vi "Read from UDP.vi"(8 "error in":errorcluster, 11 "Control Loop Cluster":T1) -> (0 "error out":errorcluster, 3 "Control Loop Cluster Out":T1)   [LabVIEW 2021, in "RT Main.lvlib"]
uses:
  RT Main.lvlib
  Control Loop Cluster.ctl
  <vilib>/myRIO/Instrument Drivers/Onboard IO/AI/typedefs/AI Reference.ctl
  <vilib>/myRIO/Common/Instrument Driver Framework/Utilities/typedefs/myRIO Generic Hardware Reference.ctl
  <vilib>/myRIO/Common/Instrument Driver Framework/Utilities/typedefs/Hardware Version Enum.ctl
  <vilib>/myRIO/Common/Instrument Driver Framework/Utilities/typedefs/myRIO v1.0 Reference.ctl
  <vilib>/myRIO/Common/Instrument Driver Framework/Utilities/typedefs/Generic FPGA Reference.ctl
  <vilib>/myRIO/Common/Instrument Driver Framework/myRIO v1.0/AI/typedefs/AI Channels List.ctl
  <vilib>/myRIO/Common/Instrument Driver Framework/myRIO v1.0/AI/typedefs/AI Channels Enum.ctl
  <vilib>/myRIO/Common/Instrument Driver Framework/Utilities/typedefs/Analog Scaling Constants List.ctl
  <vilib>/myRIO/Common/Instrument Driver Framework/Utilities/typedefs/Analog Scaling Constants.ctl
  <vilib>/myRIO/Instrument Drivers/Onboard IO/DIO/typedefs/DIO Reference.ctl
  <vilib>/myRIO/Common/Instrument Driver Framework/myRIO v1.0/DIO/typedefs/DIO Channels List.ctl
  <vilib>/myRIO/Common/Instrument Driver Framework/myRIO v1.0/DIO/typedefs/DIO Channels Enum.ctl
  Data Cluster.ctl
  Libraries/Common RT/Hardware Monitoring.ctl
  <vilib>/myRIO/Instrument Drivers/Onboard IO/AI/AI.lvlib
  <vilib>/myRIO/Instrument Drivers/Onboard IO/DIO/DIO.lvlib
  Libraries/Common RT/Common RT.lvlib
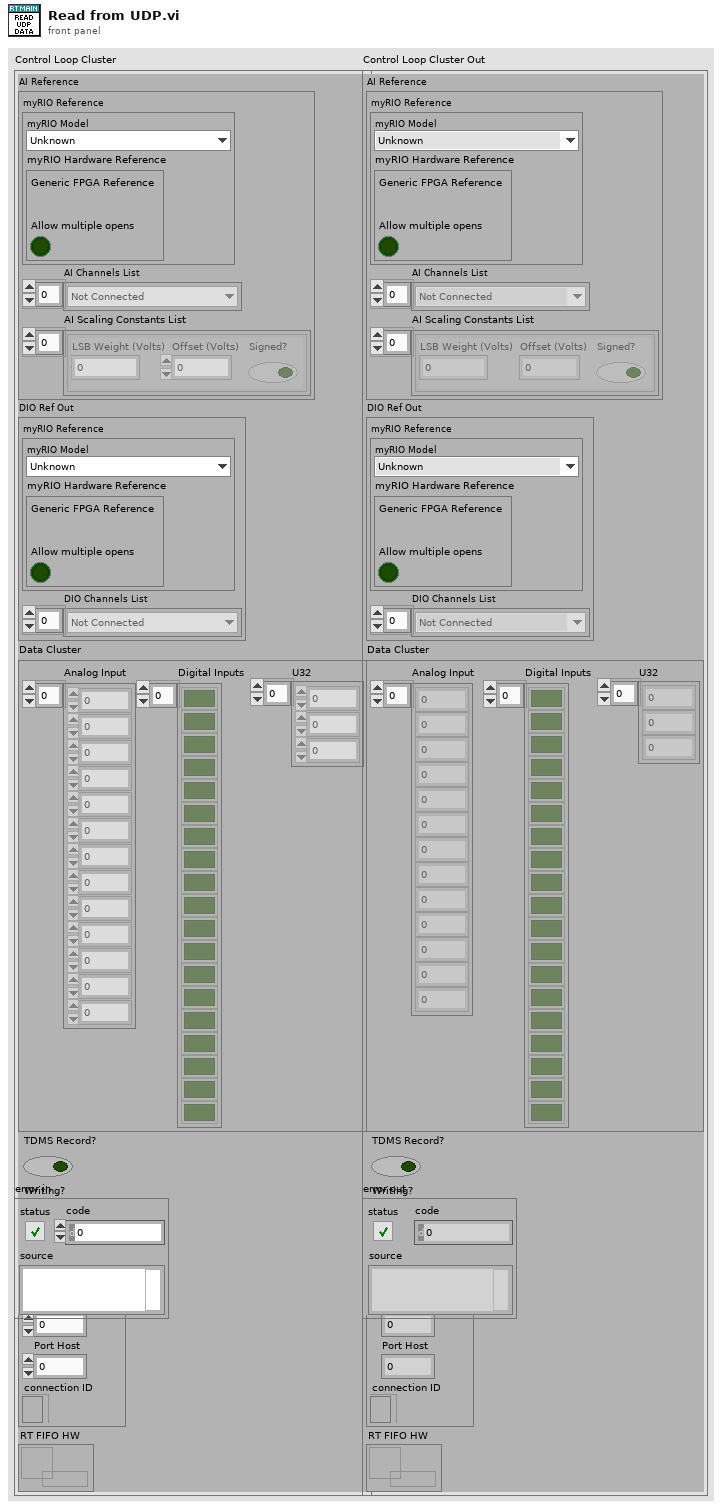
[diagram p1: front panel]
types:
  T1 = typedef "RT Main.lvlib/Control Loop Cluster.ctl" = cluster{"AI Reference":T2, "DIO Reference":T11, "Data Cluster":T14, "TDMS Record?":bool, "Writing?":bool, "UDP Info":cluster{"IP Host":string, "Port RT":u16, "Port Host":u16, "connection ID":refnum<k16>}, "RT FIFO HW":refnum<k33>}
  T2 = typedef "AI.lvlib/AI Reference.ctl" = cluster{"myRIO Reference":T3, "AI Channels List":T7, "AI Scaling Constants List":T9}
  T3 = typedef "myRIO Generic Hardware Reference.ctl" = cluster{"myRIO Model":T4, "myRIO Hardware Reference":T5}
  T4 = typedef "Hardware Version Enum.ctl" = enum16{"Unknown", "myRIO-1900", "myRIO-1950", "roboRIO", "NI ELVIS RIO CM", "ELVIS III"}
  T5 = typedef "myRIO v1.0 Reference.ctl" = cluster{"Generic FPGA Reference":T6, "Allow multiple opens":bool}
  T6 = typedef "Generic FPGA Reference.ctl" = refnum<k20>
  T7 = typedef "AI Channels List.ctl" = T8[]
  T8 = typedef "AI Channels Enum.ctl" = enum16{"Not Connected", "AudioIn/Left", "AudioIn/Right", "C/AI0", "C/AI1", "A/AI0", "A/AI1", "A/AI2", "A/AI3", "A/AI4", "A/AI5", "A/AI6", "A/AI7", "B/AI0", "B/AI1", "B/AI2", "B/AI3", "B/AI4", "B/AI5", "B/AI6", "B/AI7", "AI/AI0", "AI/AI1", "AI/AI2", "AI/AI3", "A/AI0 (DIFF)", "A/AI1 (DIFF)", "A/AI2 (DIFF)", "A/AI3 (DIFF)", "B/AI0 (DIFF)", "B/AI1 (DIFF)", "B/AI2 (DIFF)", "B/AI3 (DIFF)"}
  T9 = typedef "Analog Scaling Constants List.ctl" = T10[]
  T10 = typedef "Analog Scaling Constants.ctl" = cluster{"LSB Weight (Volts)":dbl, "Offset (Volts)":dbl, "Signed?":bool}
  T11 = typedef "DIO.lvlib/DIO Reference.ctl" = cluster{"myRIO Reference":T3, "DIO Channels List":T12}
  T12 = typedef "DIO Channels List.ctl" = T13[]
  T13 = typedef "DIO Channels Enum.ctl" = enum16{"Not Connected", "C/DIO0", "C/DIO1", "C/DIO2", "C/DIO3", "C/DIO4", "C/DIO5", "C/DIO6", "C/DIO7", "A/DIO0", "A/DIO1", "A/DIO2", "A/DIO3", "A/DIO4", "A/DIO5", "A/DIO6", "A/DIO7", "A/DIO8", "A/DIO9", "A/DIO10", "A/DIO11", "A/DIO12", "A/DIO13", "A/DIO14", "A/DIO15", "A/DIO16", "A/DIO17", "A/DIO18", "A/DIO19", "B/DIO0", "B/DIO1", "B/DIO2", "B/DIO3", "B/DIO4", "B/DIO5", "B/DIO6", "B/DIO7", "B/DIO8", "B/DIO9", "B/DIO10", "B/DIO11", "B/DIO12", "B/DIO13", "B/DIO14", "B/DIO15", "B/DIO16", "B/DIO17", "B/DIO18", "B/DIO19", "LED0", "LED1", "LED2", "LED3", "Button0", "DIO/DIO0", "DIO/DIO1", "DIO/DIO2", "DIO/DIO3", "DIO/DIO4", "DIO/DIO5", "DIO/DIO6", "DIO/DIO7", "DIO/DIO8", "DIO/DIO9", "SPI/CS0", "SPI/CS1", "SPI/CS2", "SPI/CS3", "LED RADIO (Green)", "LED RADIO (Red)", "LED COMM (Green)", "LED COMM (Red)", "LED MODE (Green)", "LED MODE (Red)"}
  T14 = typedef "RT Main.lvlib/Data Cluster.ctl" = cluster{"Analog Input":dbl[], "Digital Inputs":bool[], "U32":u32[]}
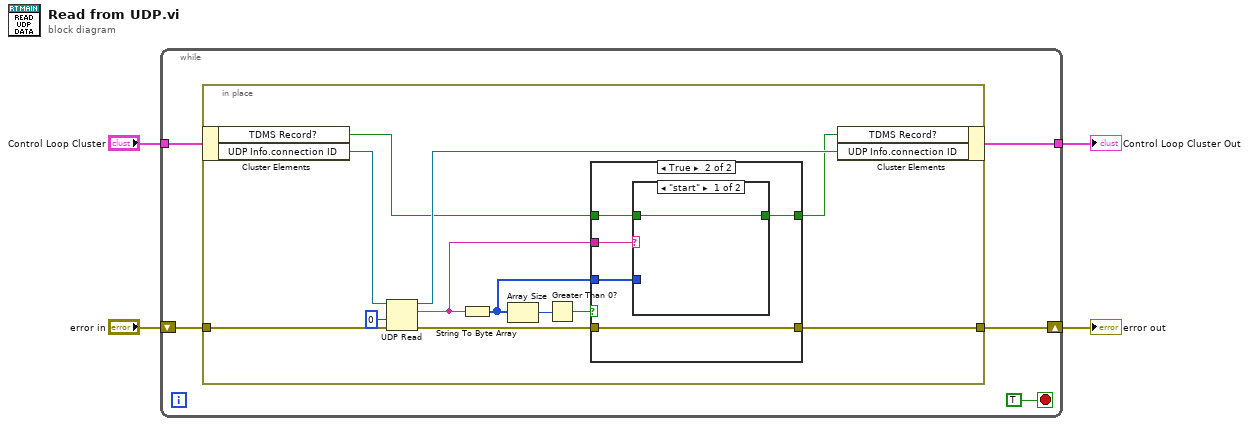
[diagram p0: block diagram]
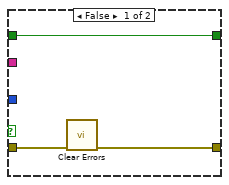
[diagram p2: hidden frame]
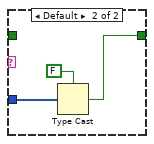
[diagram p3: hidden frame]
diagram:
  n1 = while {
    tunnel: "Control Loop Cluster" -> [w9]
    tunnel: [w7] -> w2
    shift-right: [w5] -> w1
    shift-left: "error in" -> [w8]
    stop <- TRUE stop-if-true
    n2 = in-place {
      in-place-border: w8 -> [w21]
      in-place-border: [w11] -> w5
      n3 = in-place-cluster #1(w9) -> ("TDMS Record?"=w13:bool, "UDP Info.connection ID"=w20:refnum<k16>)
      n4 = UDP Read(connection ID=w20, timeout ms (25000)=0, 8:w21) -> (data out=w10:string, error out=w14:errorcluster, 3:w19:refnum<k16>)  [unwired: 1 in, 2 out]
      n5 = String To Byte Array(string=w10) -> (unsigned byte array=w15:u8[])
      n6 = Array Size(array=w15) -> (size(s)=w17:i32)
      n7 = Greater Than 0?(x=w17) -> (x > 0?=w16:bool)
      n8 = case shown="True" w16 {
        tunnel: w15 -> [_ w29]
        tunnel: w14 -> [w23 w27]
        tunnel: w13 -> [w24 w25]
        tunnel: [w24 w28] -> w12
        tunnel: [w22 w27] -> w11
        tunnel: w10 -> [_ w26]
        frame False {
          n9 = call <vilib>:"Clear Errors.vi"("error in (no error)"=w23) -> ("error out"=w22:errorcluster)  [unwired: 5 in, 1 out]
        }
        frame True {
          n10 = case shown="\"start\"" w26 {
            tunnel: w29 -> [_ w33]
            tunnel: [w30 w31] -> w28
            tunnel: w25 -> [w30 _]
            frame "start" {
            }
            frame Default {
              n11 = Type Cast(type=FALSE, x=w33) -> (*(type *) &x=w31:bool)
            }
          }
        }
      }
      n12 = in-place-cluster #1("TDMS Record?"=w12, "UDP Info.connection ID"=w19) -> (w7:T1)
    }
  }
  "Control Loop Cluster Out" <- w2
  "error out" <- w1
